vi "Gamepad Control.vi"() -> ()   [LabVIEW 2013]
uses:
  <vilib>/Utility/inputDevices.llb/closeJoystick.vi
  <vilib>/Utility/inputDevices.llb/joystickAcquire.vi
panel:
  out "logx(y)":T1
  out "s? t:f 2":i32
  out "s? t:f":i32
  out "axis info":T2
  out "Polling Loop Counter":i32
  in  "Stop Button":bool
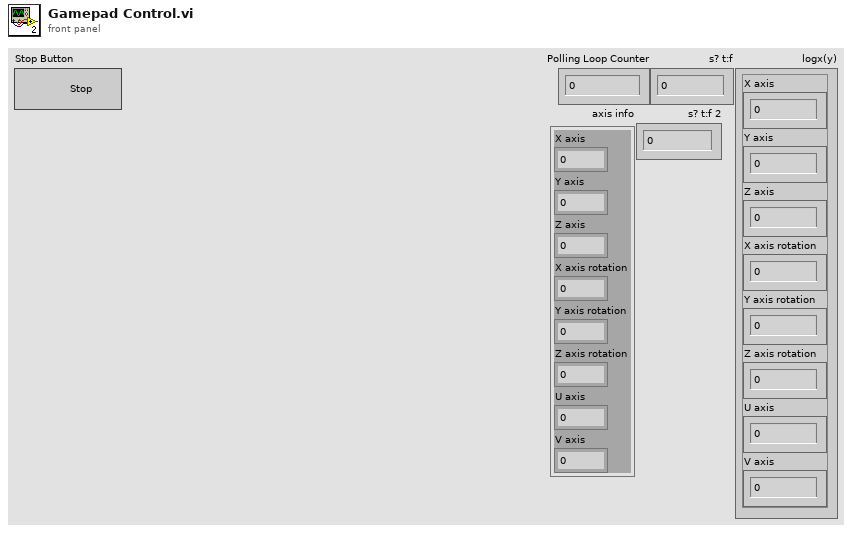
[diagram p1: front panel]
types:
  T1 = cluster{"X axis":dbl, "Y axis":dbl, "Z axis":dbl, "X axis rotation":dbl, "Y axis rotation":dbl, "Z axis rotation":dbl, "U axis":dbl, "V axis":dbl}
  T2 = cluster{"X axis":i32, "Y axis":i32, "Z axis":i32, "X axis rotation":i32, "Y axis rotation":i32, "Z axis rotation":i32, "U axis":i32, "V axis":i32}
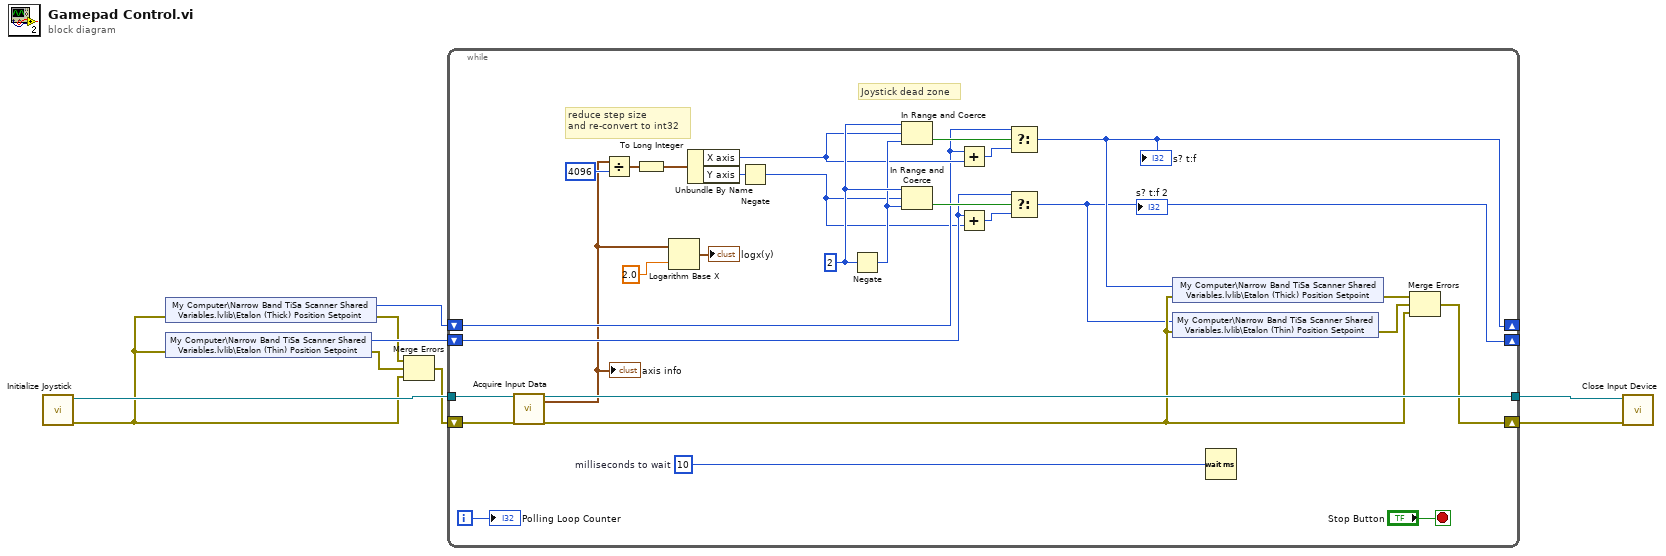
[diagram p0: block diagram]
diagram:
  n1 = call <vilib>:"Initialize Joystick.vi"() -> ("error out"=w2:errorcluster, "device ID"=w8:refnum<k1>)  [unwired: 10 in]
  n2 = shared-variable "My Computer\\Narrow Band TiSa Scanner Shared Variables.lvlib\\Etalon (Thick) Position Setpoint"(error in=w2) -> (w5:i32, error out=w4:errorcluster)
  n3 = shared-variable "My Computer\\Narrow Band TiSa Scanner Shared Variables.lvlib\\Etalon (Thin) Position Setpoint"(error in=w2) -> (w6:i32, error out=w3:errorcluster)
  n4 = Merge Errors(w4, w3, w2) -> (w1:errorcluster)
  n5 = while {
    shift-right: [w27] -> w9
    shift-left: w1 -> [w36]
    tunnel: w8 -> [w35]
    tunnel: [w34] -> w7
    shift-right: [w11] -> _
    shift-left: w6 -> [w19]
    shift-right: [w12] -> _
    shift-left: w5 -> [w16]
    i -> [w37]
    stop <- "Stop Button" stop-if-true
    w25 = 2
    w33 = u32 10  # milliseconds to wait
    # "Joystick dead zone"
    # "reduce step size\nand re-convert to int32"
    n6 = call-poly <vilib>:"Acquire Input Data.vi"("device ID"=w35, "error in (no error)"=w36) -> ("device ID"=w34:refnum<k1>, "axis info"=w15:T2, "error out"=w28:errorcluster)  [unwired: 13 in, 2 out]
    "axis info" <- w15
    n7 = Divide(x=w15, y=4096) -> (x/y=w31:T1)
    n8 = To Long Integer(number=w31) -> (32bit integer=w26:T2)
    n9 = Logarithm Base X(1:2.0, 2:w15) -> (0:→"logx(y)":T1)
    n10 = Unbundle By Name(w26) -> ("X axis"=w18:i32, "Y axis"=w17:i32)
    n11 = Negate(x=w17) -> (-x=w10:i32)
    n12 = Negate(x=w25) -> (-x=w24:i32)
    n13 = In Range and Coerce(upper limit=w25, x=w18, lower limit=w24) -> (In Range?=w23:bool)  [unwired: 1 out]
    n14 = In Range and Coerce(upper limit=w25, x=w10, lower limit=w24) -> (In Range?=w22:bool)  [unwired: 1 out]
    n15 = Add(x=w16, y=w18) -> (x+y=w21:i32)
    n16 = Add(x=w19, y=w10) -> (x+y=w20:i32)
    n17 = Select(t=w16, s=w23, f=w21) -> (s? t:f=w12:i32)
    "s? t:f" <- w12
    n18 = Select(t=w19, s=w22, f=w20) -> (s? t:f=w11:i32)
    "s? t:f 2" <- w11
    n19 = shared-variable "My Computer\\Narrow Band TiSa Scanner Shared Variables.lvlib\\Etalon (Thick) Position Setpoint"(w12, error in=w28) -> (error out=w30:errorcluster)
    n20 = shared-variable "My Computer\\Narrow Band TiSa Scanner Shared Variables.lvlib\\Etalon (Thin) Position Setpoint"(w11, error in=w28) -> (error out=w29:errorcluster)
    n21 = Wait (ms)(milliseconds to wait=w33) -> ()  [unwired: 1 out]
    n22 = Merge Errors(w30, w29, w28) -> (w27:errorcluster)
    "Polling Loop Counter" <- w37
  }
  n23 = call-poly <vilib>:"Close Input Device.vi"("error in (no error)"=w9, "device ID"=w7) -> ()  [unwired: 8 in, 1 out]
